vi "Set all channels Mean.vi"(8 "error in (no error)":errorcluster, 10 "Boolean":bool=TRUE, 11 "Graph Manager in":refnum<class "Graph Manager.lvclass">) -> (0 "error out":errorcluster, 3 "Graph Manager out":refnum<class "Graph Manager.lvclass">)   [LabVIEW 2016, in "Graph Manager.lvclass"]
uses:
  Graph Manager.lvclass
  Graph Manager.lvclass/Graph Manager.ctl
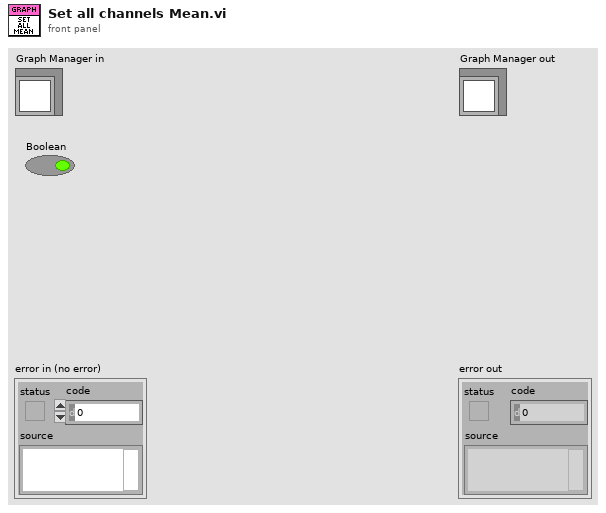
[diagram p1: front panel]
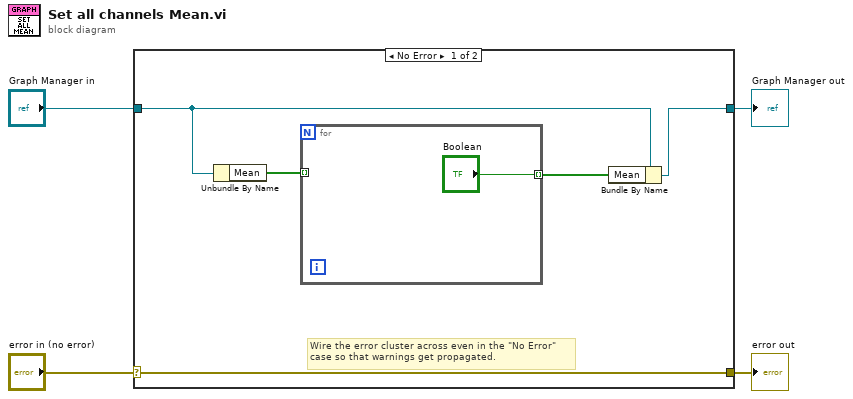
[diagram p0: block diagram]
diagram:
  n1 = case shown="No Error" "error in (no error)" {
    selector: "error in (no error)" -> [w9 w12]
    tunnel: [w9 w12] -> w3
    tunnel: [w6 w11] -> w1
    tunnel: "Graph Manager in" -> [w7 w11]
    frame No Error {
      # "Wire the error cluster across even in the \"No Error\"\ncase so that warnings get propagated."
      n2 = Unbundle By Name(w7) -> ("Mean"=w8:bool[])
      n3 = for {
        tunnel: w8 -> [_] mode=indexing
        tunnel: ["Boolean"] -> w5 mode=indexing
      }
      n4 = Bundle By Name(cluster=w7, "Mean"=w5) -> (w6:refnum<class "Graph Manager.lvclass">)
    }
    frame Error {
    }
  }
  "error out" <- w3
  "Graph Manager out" <- w1
